vi "JSONRPC-SplitArray.vi"(11 "JSON Array":string) -> (3 "Array":string[](array[string]))   [LabVIEW 2014]
panel:
  # "SplitArray"
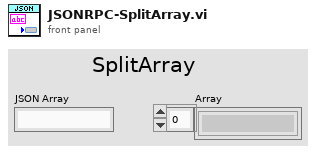
[diagram p1: front panel]
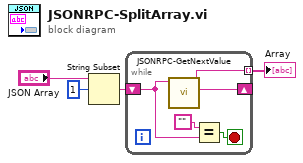
[diagram p0: block diagram]
diagram:
  n1 = String Subset(string="JSON Array", offset (0)=1) -> (substring=w1:string)  [unwired: 1 in]
  n2 = while {
    shift-right: [w9] -> _
    shift-left: w1 -> [w7]
    tunnel: [w5] -> w4 mode=indexing
    stop <- w8 stop-if-true
    n3 = call "JSONRPC-GetNextValue.vi"("Input"=w7) -> ("Rest"=w9:string, "Next"=w5:string)  [unwired: 9 in]
    n4 = Equal?(x="", y=w7) -> (x = y?=w8:bool)
  }
  "Array" <- w4
